vi "Tell Reply.vi"(4 "Priority":bool, 6 "Teller":refnum<class "Teller.lvclass">, 7 "Actor in":refnum<class "Actor.lvclass">, 8 "Error in":errorcluster) -> (0 "Error out":errorcluster, 5 "Actor out":refnum<class "Actor.lvclass">)   [LabVIEW 2025, in "_Template.lvlib" / "Templates.lvlib" / "TEMPLATE jettl Msg.lvlib" / "TEMPLATE.lvlib"]
uses:
  TEMPLATE.lvlib
  jettl/jettl/Teller/Teller.lvclass
  jettl/jettl/Actor/Actor.lvclass
  Init Msg.vi
  jettl/jettl/jettl.lvlib
panel:
  # "This front panel should not be manipulated."
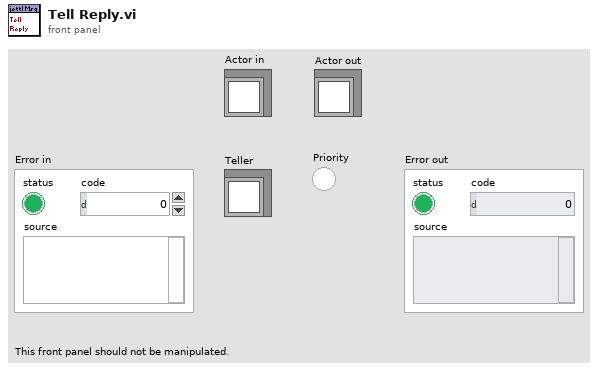
[diagram p1: front panel]
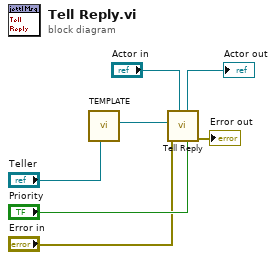
[diagram p0: block diagram]
diagram:
  n1 = call-poly "TEMPLATE.vi"("Teller"="Teller") -> ("Msg"=w3:refnum<class "Msg.lvclass">)  [unwired: 10 in]
  n2 = call "Tell Reply.vi"("Priority"="Priority", "Actor in"="Actor in", "Error in"="Error in", "Msg"=w3) -> ("Error out"=→"Error out":errorcluster, "Actor out"=→"Actor out":refnum<class "Actor.lvclass">)  [unwired: 6 in]
